vi "MakeGradualChangeColorBar.vi"(1 "FalseColorData":T1, 2 "Direction":enum16{"Horizontal", "Vertical"}(ring), 3 "GradualChangeColorBar Size":T2) -> (0 "GradualChangeColorBarPicDat":u32[][](array[numeric]))   [LabVIEW 2016]
uses:
  <vilib>/Utility/miscctls.llb/LVBoundsTypeDef.ctl
panel:
  # "This VI is to draw a gradual change color bar according to  false color"
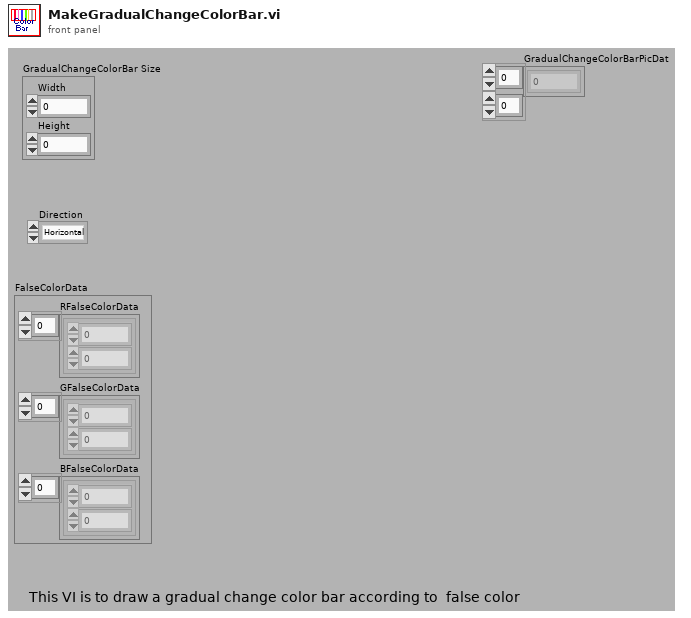
[diagram p1: front panel]
types:
  T1 = cluster{"RFalseColorData":cluster{dbl, dbl}[], "GFalseColorData":cluster{dbl, dbl}[], "BFalseColorData":cluster{dbl, dbl}[]}
  T2 = typedef "LVBoundsTypeDef.ctl" = cluster{"Width":u32, "Height":u32}
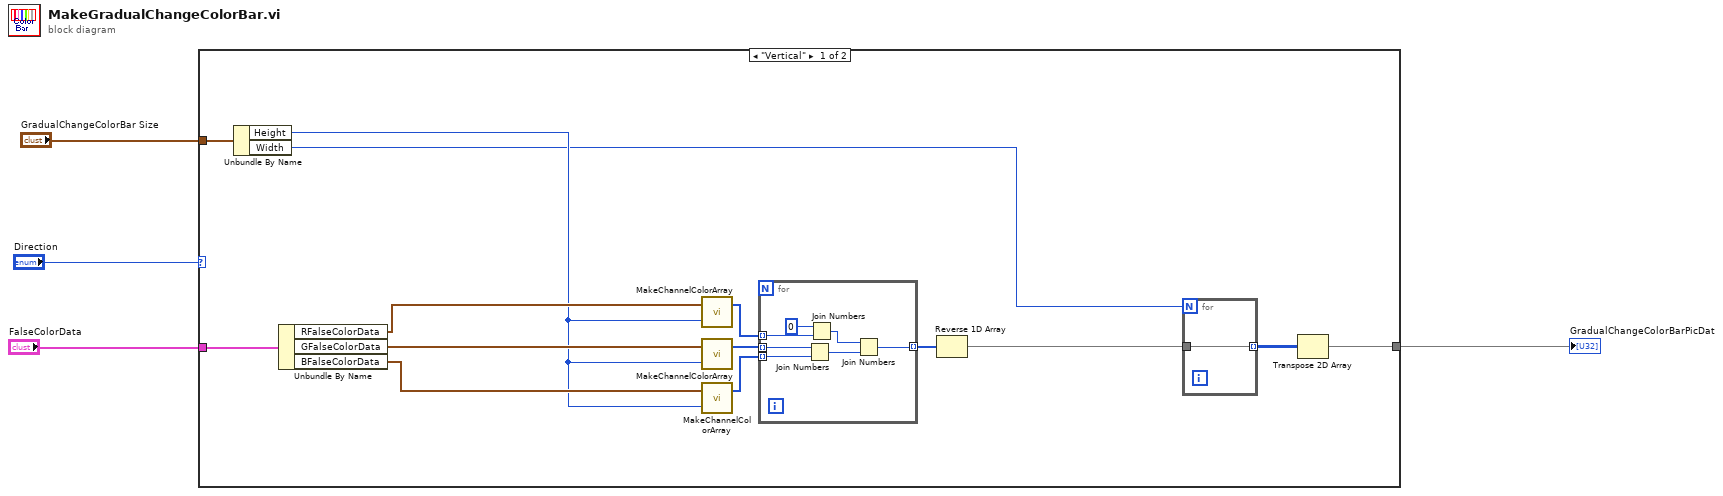
[diagram p0: block diagram]
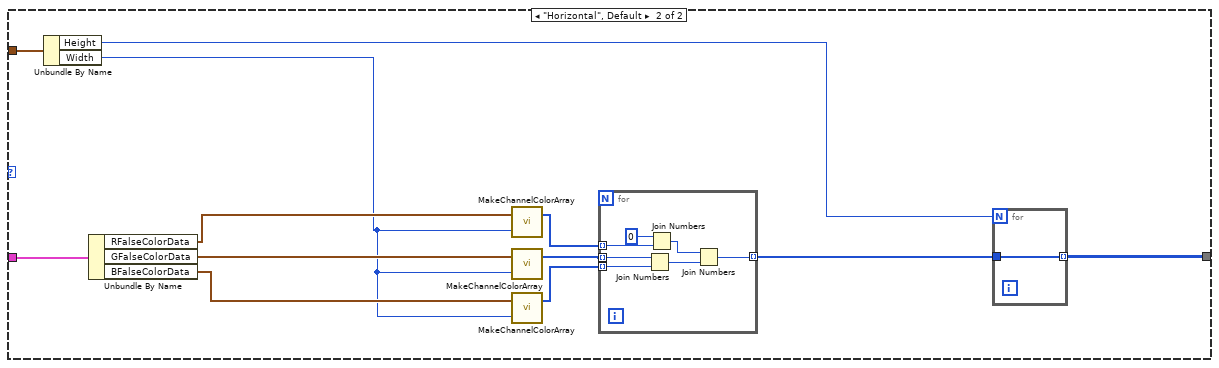
[diagram p2: hidden frame]
diagram:
  n1 = case shown="\"Vertical\"" "Direction" {
    tunnel: "FalseColorData" -> [w15 w38]
    tunnel: "GradualChangeColorBar Size" -> [w12 w35]
    tunnel: [w6 w32] -> w2
    frame "Vertical" {
      n2 = Unbundle By Name(w12) -> ("Height"=w10:u32, "Width"=w7:u32)
      n3 = Unbundle By Name(w15) -> ("RFalseColorData"=w11:cluster{dbl, dbl}[], "GFalseColorData"=w14:cluster{dbl, dbl}[], "BFalseColorData"=w13:cluster{dbl, dbl}[])
      n4 = call "MakeChannelColorArray.vi"("ArrayLength"=w10, "FalseColorDat"=w11) -> ("GradualChangeColorBar1DArray"=w16:u8[])  [unwired: 1 out]
      n5 = call "MakeChannelColorArray.vi"("ArrayLength"=w10, "FalseColorDat"=w14) -> ("GradualChangeColorBar1DArray"=w18:u8[])  [unwired: 1 out]
      n6 = call "MakeChannelColorArray.vi"("ArrayLength"=w10, "FalseColorDat"=w13) -> ("GradualChangeColorBar1DArray"=w17:u8[])  [unwired: 1 out]
      n7 = for {
        tunnel: w16 -> [w23] mode=indexing
        tunnel: w18 -> [w21] mode=indexing
        tunnel: w17 -> [w20] mode=indexing
        tunnel: [w22] -> w8 mode=indexing
        n8 = Join Numbers(hi=w21, lo=w20) -> ((hi.lo)=w25:u16)
        n9 = Join Numbers(hi=u8 0, lo=w23) -> ((hi.lo)=w26:u16)
        n10 = Join Numbers(hi=w26, lo=w25) -> ((hi.lo)=w22:u32)
      }
      n11 = Reverse 1D Array(array=w8) -> (reversed array=w9:u32[])
      n12 = for {
        N: w7 -> [_]
        tunnel: w9 -> [w19]
        tunnel: [w19] -> w5 mode=indexing
      }
      n13 = Transpose 2D Array(2D array=w5) -> (transposed array=w6:u32[][])
    }
    frame "Horizontal", Default {
      n14 = Unbundle By Name(w35) -> ("Height"=w33:u32, "Width"=w31:u32)
      n15 = Unbundle By Name(w38) -> ("RFalseColorData"=w34:cluster{dbl, dbl}[], "GFalseColorData"=w37:cluster{dbl, dbl}[], "BFalseColorData"=w36:cluster{dbl, dbl}[])
      n16 = call "MakeChannelColorArray.vi"("ArrayLength"=w31, "FalseColorDat"=w34) -> ("GradualChangeColorBar1DArray"=w29:u8[])  [unwired: 1 out]
      n17 = call "MakeChannelColorArray.vi"("ArrayLength"=w31, "FalseColorDat"=w37) -> ("GradualChangeColorBar1DArray"=w28:u8[])  [unwired: 1 out]
      n18 = call "MakeChannelColorArray.vi"("ArrayLength"=w31, "FalseColorDat"=w36) -> ("GradualChangeColorBar1DArray"=w27:u8[])  [unwired: 1 out]
      n19 = for {
        tunnel: w29 -> [w42] mode=indexing
        tunnel: w28 -> [w40] mode=indexing
        tunnel: w27 -> [w39] mode=indexing
        tunnel: [w41] -> w30 mode=indexing
        n20 = Join Numbers(hi=w40, lo=w39) -> ((hi.lo)=w44:u16)
        n21 = Join Numbers(hi=u8 0, lo=w42) -> ((hi.lo)=w45:u16)
        n22 = Join Numbers(hi=w45, lo=w44) -> ((hi.lo)=w41:u32)
      }
      n23 = for {
        N: w33 -> [_]
        tunnel: w30 -> [w46]
        tunnel: [w46] -> w32 mode=indexing
      }
    }
  }
  "GradualChangeColorBarPicDat" <- w2
